vi "sv_Compute RMS Overall Level.vi"(7 "reset":bool, 8 "integration revolution":u32=1, 10 "even angle position info in":T1, 11 "even angle signals":cluster{"r0":dbl, "dr":dbl, "Y":dbl[]}[](array[cluster])) -> (0 "output length":i32, 1 "decimation factor":i32, 2 "even angle position info out":T1, 3 "output RMS level":dbl[][](array[numeric]))   [LabVIEW 2017, in "SoundVib_ContSweptSine.lvlib"]
uses:
  <vilib>/addons/Sound and Vibration/svt_Continuous Swept Sine/SoundVib_ContSweptSine.lvlib
  <vilib>/addons/Sound and Vibration/Order Analysis/Misc/OAT Position Info.ctl
  <vilib>/Analysis/5stat.llb/RMS (DBL).vi
  <vilib>/Analysis/NI_AALPro.lvlib
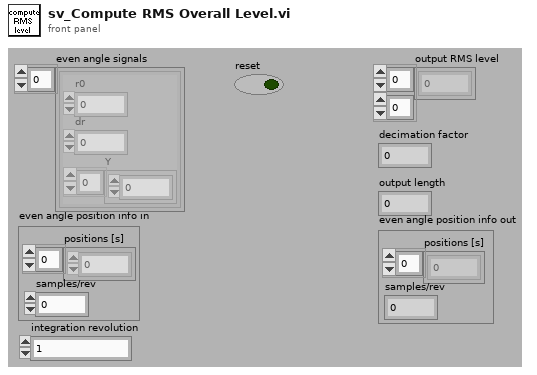
[diagram p1: front panel]
types:
  T1 = typedef "OAT Position Info.ctl" = cluster{"positions [s]":dbl[], "samples/rev":dbl}
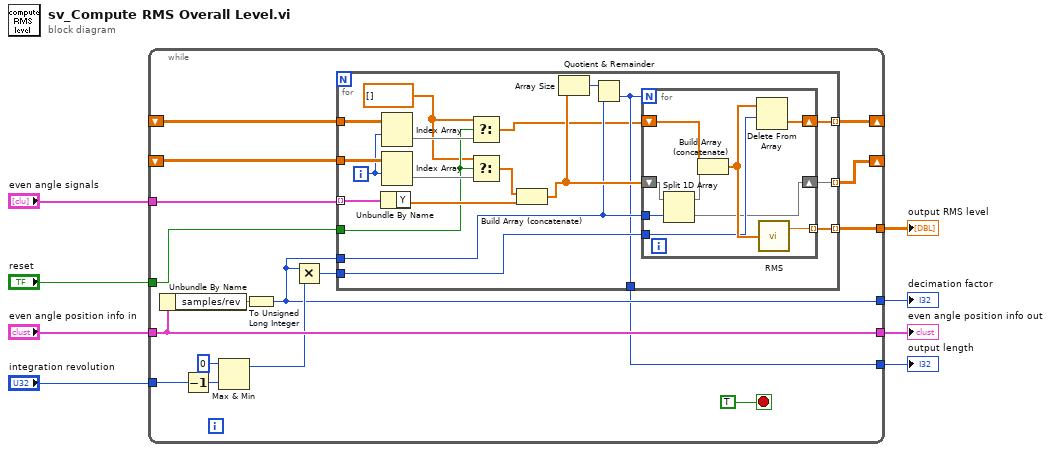
[diagram p0: block diagram]
diagram:
  n1 = while {
    tunnel: "integration revolution" -> [w21]
    tunnel: "even angle signals" -> [w10]
    tunnel: "reset" -> [w9]
    shift-right: [w24] -> _
    shift-left: _ -> [w12]
    tunnel: "even angle position info in" -> [w22]
    tunnel: [w23] -> w7
    tunnel: [w16] -> w8
    tunnel: [w14] -> w6
    tunnel: [w22] -> w1
    shift-right: [w13] -> _
    shift-left: _ -> [w11]
    stop <- TRUE stop-if-true
    n2 = Unbundle By Name(w22) -> ("samples/rev"=w20:dbl)
    n3 = Decrement(x=w21) -> (x-1=w19:u32)
    n4 = Max & Min(x=u32 0, y=w19) -> (max(x,y)=w18:u32)  [unwired: 1 out]
    n5 = To Unsigned Long Integer(number=w20) -> (unsigned 32bit integer=w16:u32)
    n6 = Multiply(x=w16, y=w18) -> (x*y=w15:u32)
    n7 = for {
      tunnel: [w38] -> w24 mode=indexing
      tunnel: [w37] -> w23 mode=indexing
      tunnel: w16 -> [w40]
      tunnel: w10 -> [w44] mode=indexing
      tunnel: w15 -> [w43]
      tunnel: [w39] -> w14
      tunnel: [w36] -> w13 mode=indexing
      tunnel: w11 -> [w35]
      tunnel: w12 -> [w34]
      tunnel: w9 -> [w28]
      i -> [w33]
      w27 = dbl[] [] ("t")
      n8 = Unbundle By Name(w44) -> ("Y"=w32:dbl[])
      n9 = Index Array(array=w34, index (row)=w33) -> (element=w31:dbl[])  [unwired: 1 in]
      n10 = Index Array(array=w35, index (row)=w33) -> (element=w29:dbl[])  [unwired: 1 in]
      n11 = Select(t=w27, s=w28, f=w31) -> (s? t:f=w30:dbl[])
      n12 = Select(t=w27, s=w28, f=w29) -> (s? t:f=w26:dbl[])
      n13 = Build Array (concatenate)(w26, w32) -> (w42:dbl[])
      n14 = Array Size(array=w42) -> (size(s)=w41:i32)
      n15 = Quotient & Remainder(x=w41, y=w40) -> (floor(x/y)=w39:u32)  [unwired: 1 out]
      n16 = for {
        N: w39 -> [_]
        shift-right: [w45] -> w36
        shift-left: w42 -> [w53]
        shift-right: [w48] -> w38
        shift-left: w30 -> [w51]
        tunnel: w40 -> [w52]
        tunnel: w43 -> [w49]
        tunnel: [w47] -> w37 mode=indexing
        n17 = Split 1D Array(array=w53, index=w52) -> (first subarray=w46:dbl[], second subarray=w45:dbl[])
        n18 = Build Array (concatenate)(w51, w46) -> (w50:dbl[])
        n19 = Delete From Array(array=w50, length=w49) -> (deleted portion=w48:dbl[])  [unwired: 1 in, 1 out]
        n20 = call-poly <vilib>:"RMS.vi"("X"=w50) -> ("rms value"=w47:dbl)  [unwired: 1 out]
      }
    }
  }
  "decimation factor" <- w8
  "output RMS level" <- w7
  "output length" <- w6
  "even angle position info out" <- w1
